vi "Project2FrontPanel.vi"() -> ()   [LabVIEW 2018]
uses:
  StateVariable.ctl
panel:
  in  "Code Entry Buttons":bool[](array[boolean])
  in  "Reset":bool
  out "State":T1
  out "Clock":bool
  in  "STOP":bool
  out "Lock \nStatus":bool[](array[boolean])
  # "B0"
  # "Locked"
  # "C"
  # "B"
  # "B1"
  # "A"
  # "B2"
  # "B3"
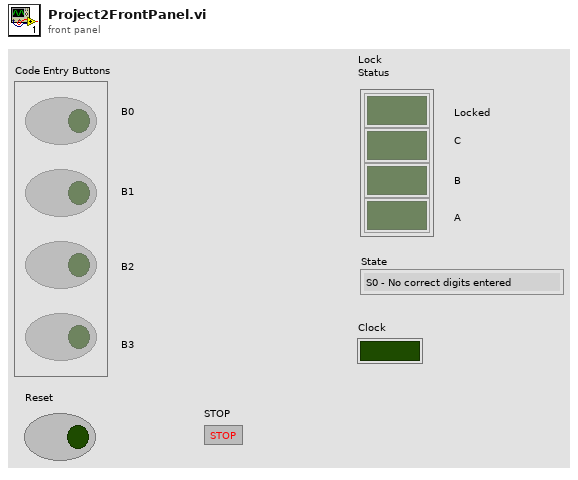
[diagram p1: front panel]
types:
  T1 = typedef "StateVariable.ctl" = enum16{"S0 - No correct digits entered", "S1 - One correct digit entered", "S2 - Two correct digits entered", "S3 - Three correct digits entered.", "S4 - Code entered"}
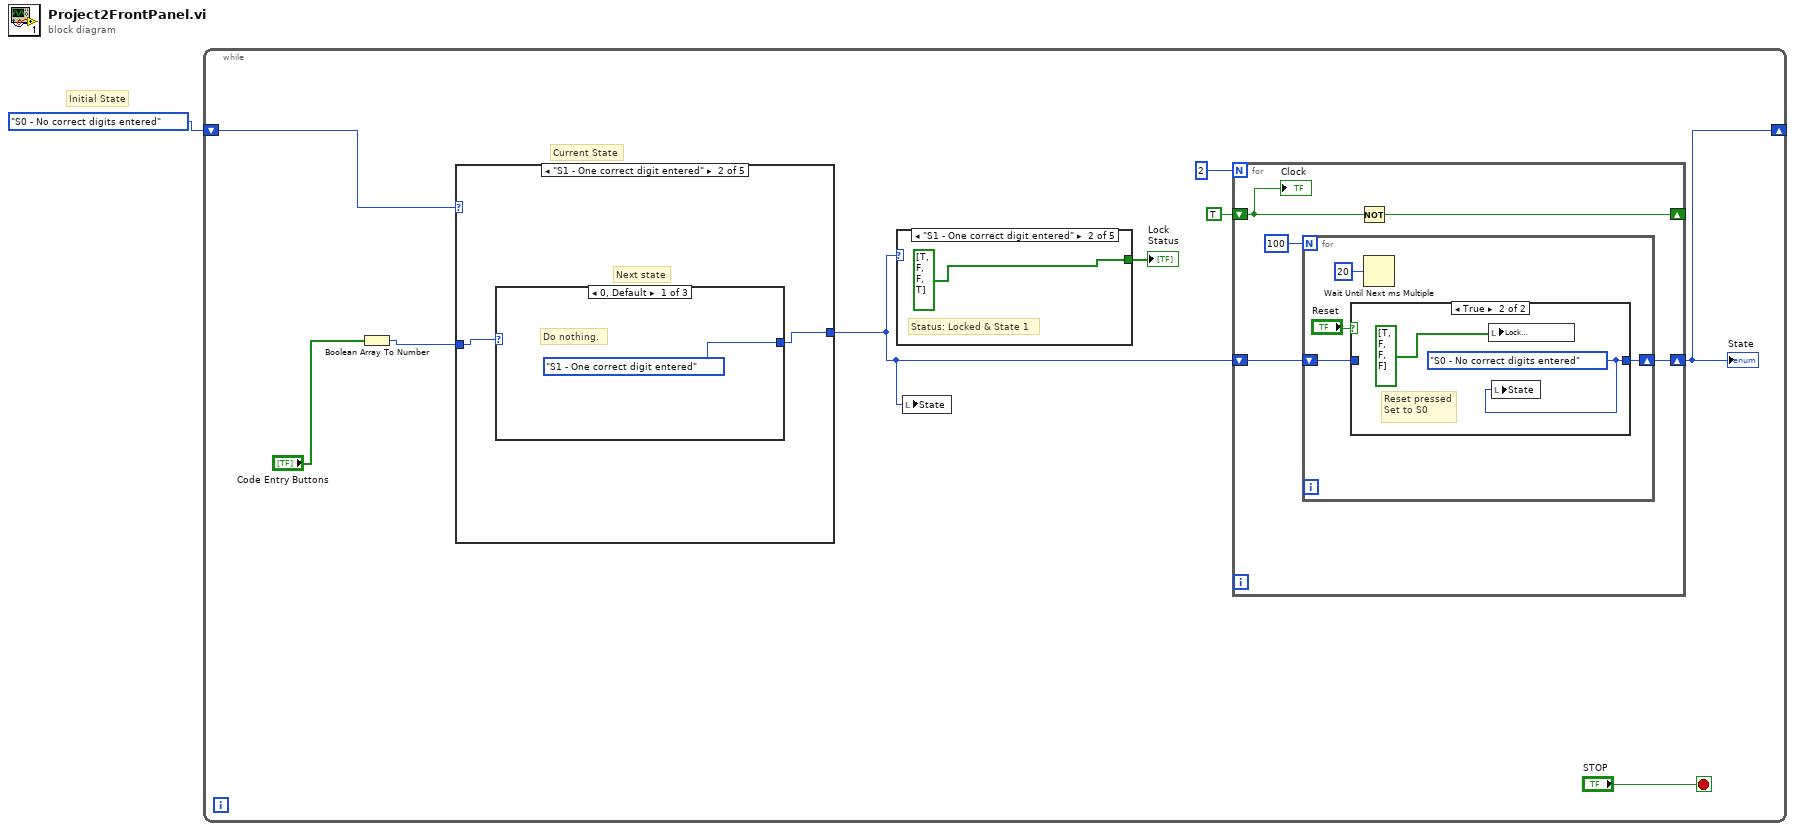
[diagram p0: block diagram]
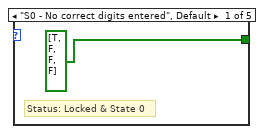
[diagram p2: hidden frame]
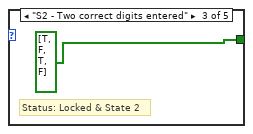
[diagram p3: hidden frame]
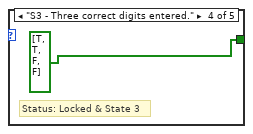
[diagram p4: hidden frame]
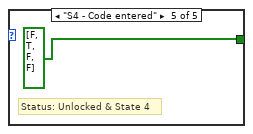
[diagram p5: hidden frame]
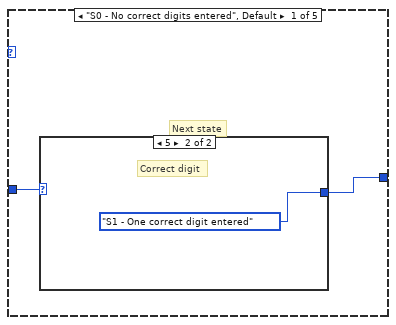
[diagram p6: hidden frame]
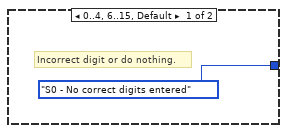
[diagram p7: hidden frame]
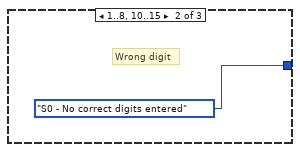
[diagram p8: hidden frame]
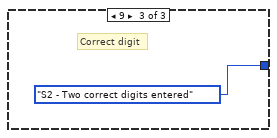
[diagram p9: hidden frame]
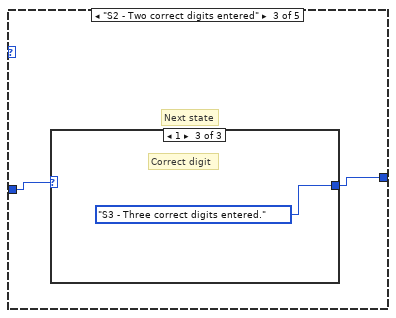
[diagram p10: hidden frame]
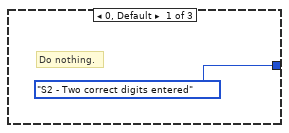
[diagram p11: hidden frame]
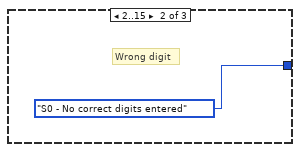
[diagram p12: hidden frame]
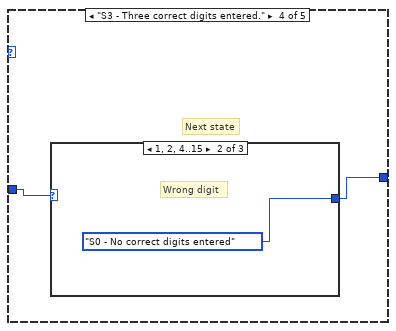
[diagram p13: hidden frame]
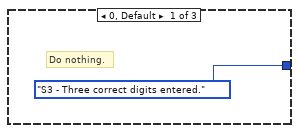
[diagram p14: hidden frame]
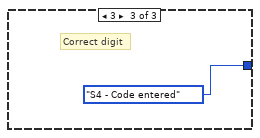
[diagram p15: hidden frame]
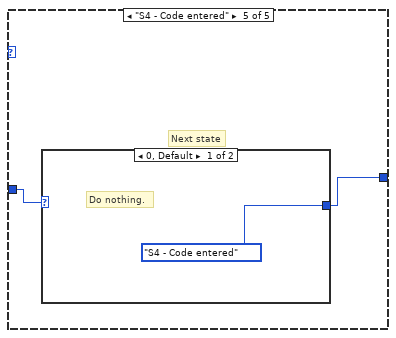
[diagram p16: hidden frame]
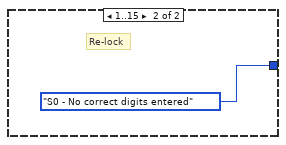
[diagram p17: hidden frame]
diagram:
  # "Initial State"
  n1 = while {
    shift-right: [w7] -> _
    shift-left: StateVariable."S0 - No correct digits entered" ("State") -> [w6]
    stop <- "STOP" stop-if-true
    # "Current State"
    n2 = Boolean Array To Number(Boolean array="Code Entry Buttons") -> (number=w4:u32)
    n3 = case shown="\"S1 - One correct digit entered\"" w6 {
      tunnel: [w17 w20 w25 w30 w36] -> w2
      tunnel: w4 -> [w16 w21 w26 w31 w35]
      frame "S0 - No correct digits entered", Default {
        # "Next state"
        n4 = case shown="5" w16 {
          tunnel: [StateVariable."S0 - No correct digits entered" ("State") StateVariable."S1 - One correct digit entered" ("State")] -> w17
          frame 0..4, 6..15, Default {
            # "Incorrect digit or do nothing."
          }
          frame 5 {
            # "Correct digit"
          }
        }
      }
      frame "S1 - One correct digit entered" {
        # "Next state"
        n5 = case shown="0, Default" w21 {
          tunnel: [StateVariable."S1 - One correct digit entered" ("State") StateVariable."S0 - No correct digits entered" ("State") StateVariable."S2 - Two correct digits entered" ("State")] -> w20
          frame 0, Default {
            # "Do nothing."
          }
          frame 1..8, 10..15 {
            # "Wrong digit"
          }
          frame 9 {
            # "Correct digit"
          }
        }
      }
      frame "S2 - Two correct digits entered" {
        # "Next state"
        n6 = case shown="1" w26 {
          tunnel: [StateVariable."S2 - Two correct digits entered" ("State") StateVariable."S0 - No correct digits entered" ("State") StateVariable."S3 - Three correct digits entered." ("State")] -> w25
          frame 0, Default {
            # "Do nothing."
          }
          frame 2..15 {
            # "Wrong digit"
          }
          frame 1 {
            # "Correct digit"
          }
        }
      }
      frame "S3 - Three correct digits entered." {
        # "Next state"
        n7 = case shown="1, 2, 4..15" w31 {
          tunnel: [StateVariable."S3 - Three correct digits entered." ("State") StateVariable."S0 - No correct digits entered" ("State") StateVariable."S4 - Code entered" ("State")] -> w30
          frame 0, Default {
            # "Do nothing."
          }
          frame 1, 2, 4..15 {
            # "Wrong digit"
          }
          frame 3 {
            # "Correct digit"
          }
        }
      }
      frame "S4 - Code entered" {
        # "Next state"
        n8 = case shown="0, Default" w35 {
          tunnel: [StateVariable."S4 - Code entered" ("State") StateVariable."S0 - No correct digits entered" ("State")] -> w36
          frame 0, Default {
            # "Do nothing."
          }
          frame 1..15 {
            # "Re-lock"
          }
        }
      }
    }
    n9 = case shown="\"S1 - One correct digit entered\"" w2 {
      tunnel: [bool[] [TRUE, FALSE, FALSE, FALSE] bool[] [TRUE, FALSE, FALSE, TRUE] bool[] [TRUE, FALSE, TRUE, FALSE] bool[] [TRUE, TRUE, FALSE, FALSE] bool[] [FALSE, TRUE, FALSE, FALSE]] -> w5
      frame "S0 - No correct digits entered", Default {
        # "Status: Locked & State 0"
      }
      frame "S1 - One correct digit entered" {
        # "Status: Locked & State 1"
      }
      frame "S2 - Two correct digits entered" {
        # "Status: Locked & State 2"
      }
      frame "S3 - Three correct digits entered." {
        # "Status: Locked & State 3"
      }
      frame "S4 - Code entered" {
        # "Status: Unlocked & State 4"
      }
    }
    "Lock \nStatus" <- w5
    n10 = local write "State"(w2) -> ()
    n11 = for {
      N: 2 -> [_]
      shift-right: [w42] -> _
      shift-left: TRUE -> [w41]
      shift-right: [w39] -> w7
      shift-left: w2 -> [w40]
      n12 = for {
        N: 100 -> [_]
        shift-right: [w45] -> w39
        shift-left: w40 -> [w46]
        n13 = case shown="True" "Reset" {
          tunnel: w46 -> [w48 _]
          tunnel: [w48 w50] -> w45
          frame False {
            # "Reset not pressed"
          }
          frame True {
            w50 = StateVariable."S0 - No correct digits entered" ("State")
            # "Reset pressed\nSet to S0"
            n14 = local write "Lock \nStatus"(bool[] [TRUE, FALSE, FALSE, FALSE]) -> ()
            n15 = local write "State"(w50) -> ()
          }
        }
        n16 = Wait Until Next ms Multiple(millisecond multiple=u32 20) -> ()  [unwired: 1 out]
      }
      n17 = Not(x=w41) -> (.not. x?=w42:bool)
      "Clock" <- w41
    }
    "State" <- w7
  }
